vi "Gergberg Image Manipulation v2.vi"() -> ()   [LabVIEW 2012, in "LightPipes.lvlib"]
uses:
  LightPipes.lvlib
  <vilib>/vision/NI_Vision_Development_Module.lvlib
panel:
  in  "FF Resolution  (micron/pix)":dbl=2.96
  in  "Final Resolution  (micron/pix)":dbl=2.5
  out "MF Original":cluster{"X Resolution":i32, "Y Resolution":i32}={"X Resolution"=1600, "Y Resolution"=1200}
  out "FF Original":cluster{"X Resolution":i32, "Y Resolution":i32}={"X Resolution"=640, "Y Resolution"=480}
  in  "stop":bool
  out "MF":T1(plugin-control)
  out "FF":T1(plugin-control)
  in  "Balance Energy":bool=TRUE
  in  "MF Rotate 180":bool=TRUE
  in  "MF Resolution (micron/pix)":dbl=7.38
  in  "Final Size (pix)":i32=400 step=10
  in  "Run":bool
  in  "Save MF":bool
  out "FF Current":cluster{"X Resolution":i32, "Y Resolution":i32}={"X Resolution"=400, "Y Resolution"=400}
  out "MF Current":cluster{"X Resolution":i32, "Y Resolution":i32}={"X Resolution"=400, "Y Resolution"=400}
  in  "Save FF":bool
  in  "Mid Field":path=path "C:/Users/Tri/Downloads/MidfieldFarfieldForAaron/005778 2013-02-12/Masked MF.png"
  in  "Far Field":path=path "C:/Users/Tri/Downloads/MidfieldFarfieldForAaron/005778 2013-02-12/Masked FF.png"
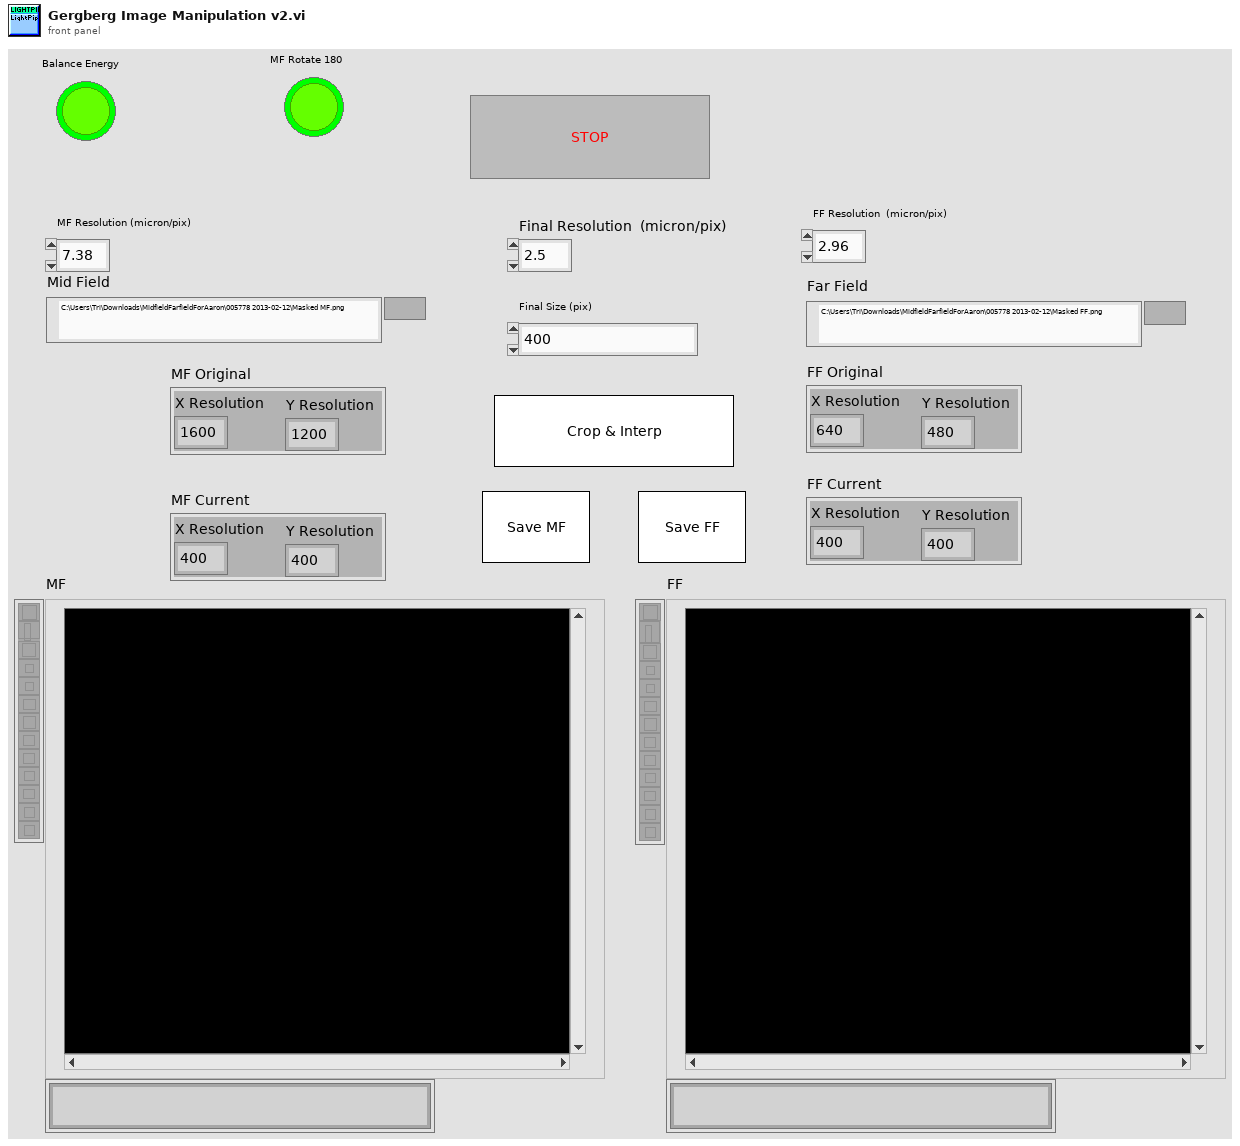
[diagram p1: front panel]
types:
  T1 = typedef "IMAQ Image.ctl" = refnum<image>
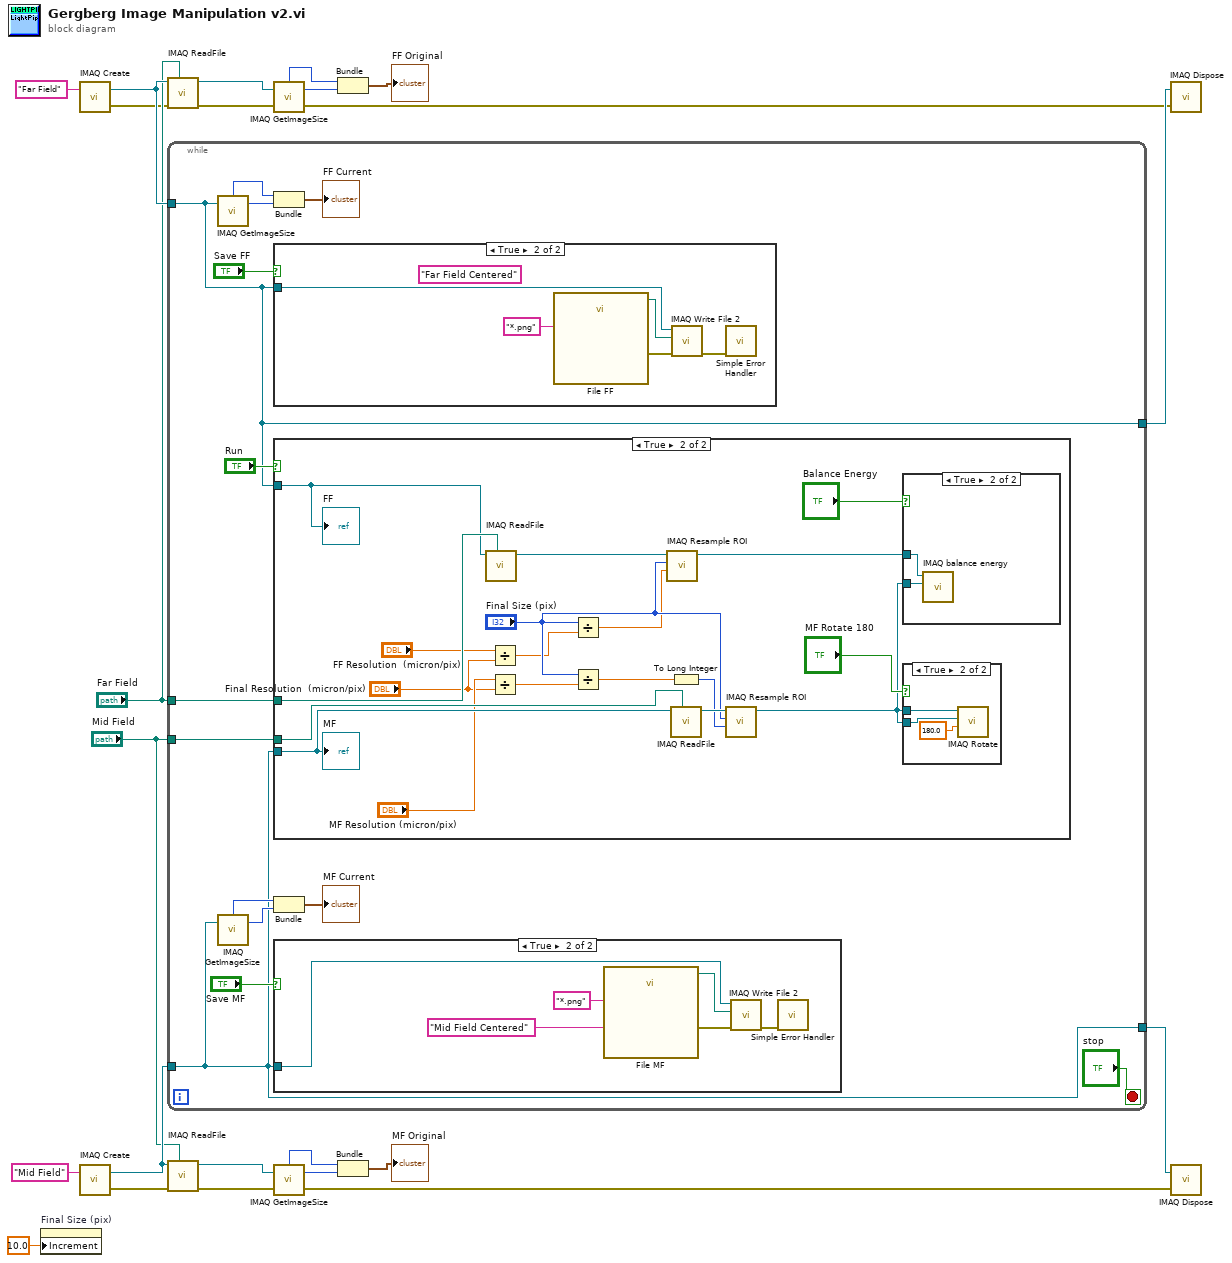
[diagram p0: block diagram]
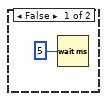
[diagram p3: hidden frame]
diagram:
  n1 = property on="Final Size (pix)" class="DigNum (strict)"("Increment"=10.0 ("Data Entry Limits:Increment")) -> ()  [unwired: 2 in, 2 out]
  n2 = call "IMAQ Create"("Image Name"="Far Field") -> ("New Image"=w20:T1, "error out"=w4:errorcluster)  [unwired: 4 in]
  n3 = call "IMAQ Create"("Image Name"="Mid Field") -> ("New Image"=w16:T1, "error out"=w2:errorcluster)  [unwired: 4 in]
  n4 = call "IMAQ ReadFile"("File Path"="Far Field", "error in (no error)"=w4, "Image"=w20) -> ("error out"=w5:errorcluster, "Image Out"=w18:T1)  [unwired: 2 in, 5 out]
  n5 = while {
    tunnel: "Far Field" -> [w36]
    tunnel: w20 -> [w24]
    tunnel: "Mid Field" -> [w35]
    tunnel: w16 -> [w26]
    tunnel: [w26] -> w8
    tunnel: [w24] -> w7
    stop <- "stop" stop-if-true
    n6 = call "IMAQ GetImageSize"("Image"=w24) -> ("Y Resolution"=w31:i32, "X Resolution"=w30:i32)  [unwired: 3 in, 1 out]
    n7 = call "IMAQ GetImageSize"("Image"=w26) -> ("Y Resolution"=w28:i32, "X Resolution"=w27:i32)  [unwired: 3 in, 1 out]
    n8 = Bundle("X Resolution"=w30, "Y Resolution"=w31) -> (→"FF Current":cluster{"X Resolution":i32, "Y Resolution":i32})  [unwired: 1 in]
    n9 = case shown="True" "Save FF" {
      tunnel: w24 -> [_ w40]
      frame False {
      }
      frame True {
        (unwired) "Far Field Centered" ("default name")
        n10 = call "File FF"("pattern (all files)"="*.png") -> ("selected path"=w42:path, "error out"=w41:errorcluster)  [unwired: 11 in, 2 out]
        n11 = call-poly "IMAQ Write File 2"("error in (no error)"=w41, "File Path"=w42, "Image"=w40) -> ("error out"=w39:errorcluster)  [unwired: 7 in, 1 out]
        n12 = call <vilib>:"Simple Error Handler.vi"("error in (no error)"=w39) -> ()  [unwired: 4 in, 5 out]
      }
    }
    n13 = case shown="True" "Run" {
      tunnel: w36 -> [_ w68]
      tunnel: w24 -> [_ w67]
      tunnel: w35 -> [_ w66]
      tunnel: w26 -> [_ w63]
      frame False {
      }
      frame True {
        n14 = call "IMAQ ReadFile"("File Path"=w68, "Image"=w67) -> ("Image Out"=w59:T1)  [unwired: 3 in, 6 out]
        n15 = Divide(x="FF Resolution  (micron/pix)", y="Final Resolution  (micron/pix)") -> (x/y=w51:dbl)
        n16 = Divide(x="MF Resolution (micron/pix)", y="Final Resolution  (micron/pix)") -> (x/y=w56:dbl)
        n17 = Divide(x="Final Size (pix)", y=w51) -> (x/y=w50:dbl)
        n18 = Divide(x="Final Size (pix)", y=w56) -> (x/y=w53:dbl)
        n19 = call "IMAQ Resample ROI.vi"("ROI Size"=w50, "Final Size"="Final Size (pix)", "Image In"=w59) -> ("Image Out"=w58:T1)  [unwired: 8 in]
        n20 = To Long Integer(number=w53) -> (32bit integer=w60:i32)
        n21 = call "IMAQ ReadFile"("File Path"=w66, "Image"=w63) -> ("Image Out"=w61:T1)  [unwired: 3 in, 6 out]
        n22 = call "IMAQ Resample ROI.vi"("ROI Size"=w60, "Final Size"="Final Size (pix)", "Image In"=w61) -> ("Image Out"=w62:T1)  [unwired: 8 in]
        n23 = case shown="True" "Balance Energy" {
          tunnel: w62 -> [_ w72]
          tunnel: w58 -> [_ w73]
          frame False {
          }
          frame True {
            n24 = call "IMAQ balance energy.vi"("Target Image"=w72, "Base Image"=w73) -> ()  [unwired: 9 in, 1 out]
          }
        }
        n25 = case shown="True" "MF Rotate 180" {
          tunnel: w62 -> [_ w70]
          tunnel: w62 -> [_ w69]
          frame False {
          }
          frame True {
            n26 = call "IMAQ Rotate"("Angle (degrees)"=sgl 180.0, "Image Dst"=w69, "Image Src"=w70) -> ()  [unwired: 7 in, 2 out]
          }
        }
        "MF" <- w63
        "FF" <- w67
      }
    }
    n27 = Bundle("X Resolution"=w27, "Y Resolution"=w28) -> (→"MF Current":cluster{"X Resolution":i32, "Y Resolution":i32})  [unwired: 1 in]
    n28 = case shown="True" "Save MF" {
      tunnel: w26 -> [_ w48]
      frame False {
        n29 = Wait (ms)(milliseconds to wait=u32 5) -> ()  [unwired: 1 out]
      }
      frame True {
        n30 = call "File MF"("prompt"="Mid Field Centered" ("default name"), "pattern (all files)"="*.png") -> ("selected path"=w49:path, "error out"=w45:errorcluster)  [unwired: 10 in, 2 out]
        n31 = call-poly "IMAQ Write File 2"("error in (no error)"=w45, "File Path"=w49, "Image"=w48) -> ("error out"=w44:errorcluster)  [unwired: 7 in, 1 out]
        n32 = call <vilib>:"Simple Error Handler.vi"("error in (no error)"=w44) -> ()  [unwired: 4 in, 5 out]
      }
    }
  }
  n33 = call "IMAQ ReadFile"("File Path"="Mid Field", "error in (no error)"=w2, "Image"=w16) -> ("error out"=w6:errorcluster, "Image Out"=w17:T1)  [unwired: 2 in, 5 out]
  n34 = call "IMAQ GetImageSize"("Image"=w18, "error in (no error)"=w5) -> ("Y Resolution"=w13:i32, "X Resolution"=w14:i32, "error out"=w3:errorcluster)  [unwired: 2 in]
  n35 = call "IMAQ GetImageSize"("Image"=w17, "error in (no error)"=w6) -> ("Y Resolution"=w9:i32, "X Resolution"=w10:i32, "error out"=w1:errorcluster)  [unwired: 2 in]
  n36 = Bundle("X Resolution"=w14, "Y Resolution"=w13) -> (→"FF Original":cluster{"X Resolution":i32, "Y Resolution":i32})  [unwired: 1 in]
  n37 = Bundle("X Resolution"=w10, "Y Resolution"=w9) -> (→"MF Original":cluster{"X Resolution":i32, "Y Resolution":i32})  [unwired: 1 in]
  n38 = call "IMAQ Dispose"("Image"=w7, "error in (no error)"=w3) -> ()  [unwired: 4 in, 1 out]
  n39 = call "IMAQ Dispose"("Image"=w8, "error in (no error)"=w1) -> ()  [unwired: 4 in, 1 out]
